vi "Clipboard.vi"() -> ()   [LabVIEW 2019]
panel:
  out "array":dbl[][](array[numeric])
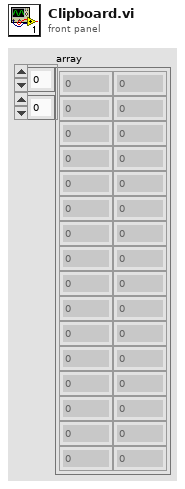
[diagram p1: front panel]
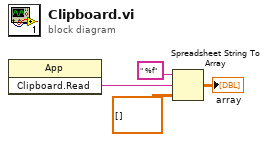
[diagram p0: block diagram]
diagram:
  n1 = invoke class="App" method="Clipboard.Read"() -> ("Read Clipbrd"=w4:string)  [unwired: 3 in, 2 out]
  n2 = Spreadsheet String To Array(format string=" %f", spreadsheet string=w4, array type (2D Dbl)=dbl[][] [] ("Array")) -> (array=→"array":dbl[][])  [unwired: 1 in]
